vi "Process Packet.vi"(8 "error in (no error)":errorcluster, 10 "Packet":string, 11 "SCADA Communications in":refnum<class "SCADA Communications.lvclass">) -> (0 "error out":errorcluster, 3 "SCADA Communications out":refnum<class "SCADA Communications.lvclass">)   [LabVIEW 2015, in "SCADA Communcations Actor.lvlib" / "SCADA Communications.lvclass"]
uses:
  SCADA Communications.lvclass
  Controls/EMS Message Cluster.ctl
  <vilib>/ActorFramework/Actor/Actor.lvclass/Actor.ctl
  SCADA Communications.lvclass/SCADA Communications.ctl
  SCADA Communications Messages/EMS Message Msg/EMS Message Msg.lvclass
  <vilib>/ActorFramework/Actor/Actor.lvclass
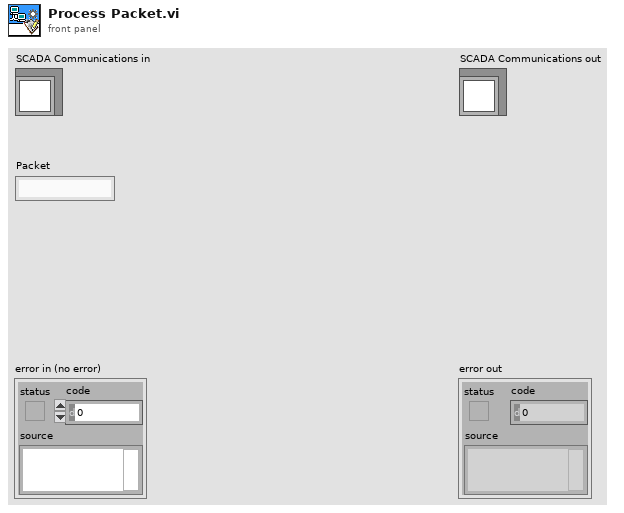
[diagram p1: front panel]
types:
  T1 = enum16{"big-endian, network order", "native, host order", "little-endian"}
  T2 = typedef "SCADA Communcations Actor.lvlib/SCADA Communications.lvclass/EMS Message Cluster.ctl" = cluster{"Name":string, "Content":string}
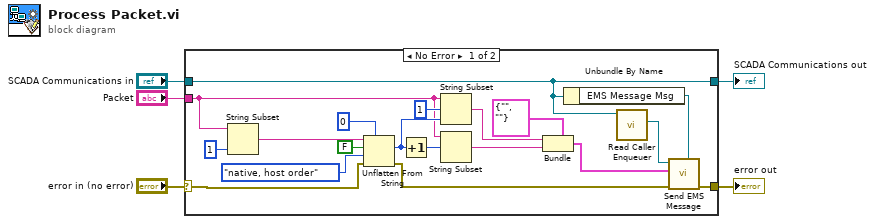
[diagram p0: block diagram]
diagram:
  n1 = case shown="No Error" "error in (no error)" {
    selector: "error in (no error)" -> [w7 w26]
    tunnel: [w22 w26] -> w4
    tunnel: [w24 w25] -> w2
    tunnel: "SCADA Communications in" -> [w24 w25]
    tunnel: "Packet" -> [w9 _]
    frame No Error {
      n2 = String Subset(string=w9, length (rest)=1 ("length (rest)")) -> (substring=w18:string)  [unwired: 1 in]
      n3 = Unflatten From String(type=u8 0, binary string=w18, data includes array or string size? (T)=FALSE, byte order (0:big-endian, network order)=T1."native, host order", error in (no error)=w7) -> (value=w16:u8, error out=w6:errorcluster)  [unwired: 1 out]
      n4 = Increment(x=w16) -> (x+1=w15:u8)
      n5 = String Subset(string=w9, offset (0)=1, length (rest)=w16) -> (substring=w13:string)
      n6 = String Subset(string=w9, offset (0)=w15) -> (substring=w12:string)  [unwired: 1 in]
      n7 = Bundle(cluster=T2 {"Name"="", "Content"=""} ("Message"), "Name"=w13, "Content"=w12) -> (w11:T2)
      n8 = Unbundle By Name(w24) -> ("EMS Message Msg"=w10:refnum<class "EMS Message Msg.lvclass">)
      n9 = call <vilib>:"Read Caller Enqueuer.vi"("Actor"=w24) -> ("Caller Enqueuer"=w23:refnum<class "Message Enqueuer.lvclass">)  [unwired: 10 in]
      n10 = call "Send EMS Message.vi"("EMS Message Msg"=w10, "error in (no error)"=w6, "Message"=w11, "Message Enqueuer in"=w23) -> ("error out"=w22:errorcluster)  [unwired: 6 in, 1 out]
    }
    frame Error {
    }
  }
  "error out" <- w4
  "SCADA Communications out" <- w2
